vi "参数设置对画框.vi"(8 "时间等比采样":u16=10, 9 "单次采样量":u16=500, 10 "采样方式":enum16{"单采", "双重"}(ring), 11 "留样模式":T1(ring)=enum."外控留样") -> ()   [LabVIEW 2016, in "超标留样集成.lvlib" / "德润DR803L超标留样.lvlib"]
uses:
  <vilib>/Utility/config.llb/NI_LVConfig.lvlib
panel:
  in  "关闭":bool
  in  "打开串口":bool
  in  "释放串口":bool
  # "只在停止时切换有效"
  # "只在待机时切换有效"
  # "默认：500ml（5-1000）ml （只在停止时写有效）"
  # "默认：10min（2-9999）min （只在停止时写有效）"
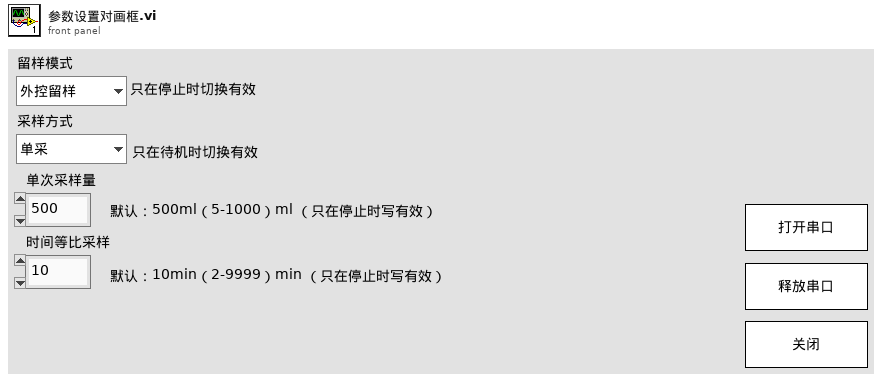
[diagram p1: front panel]
types:
  T1 = enum16{"无", "定时留样", "时间等比例", "超标留样", "同步留样", "外控留样"}
  T2 = enum16{"open", "read", "write", "write single", "close"}
  T3 = typedef "NI_LVConfig.lvlib/Config Data RefNum.ctl" = refnum<k1>
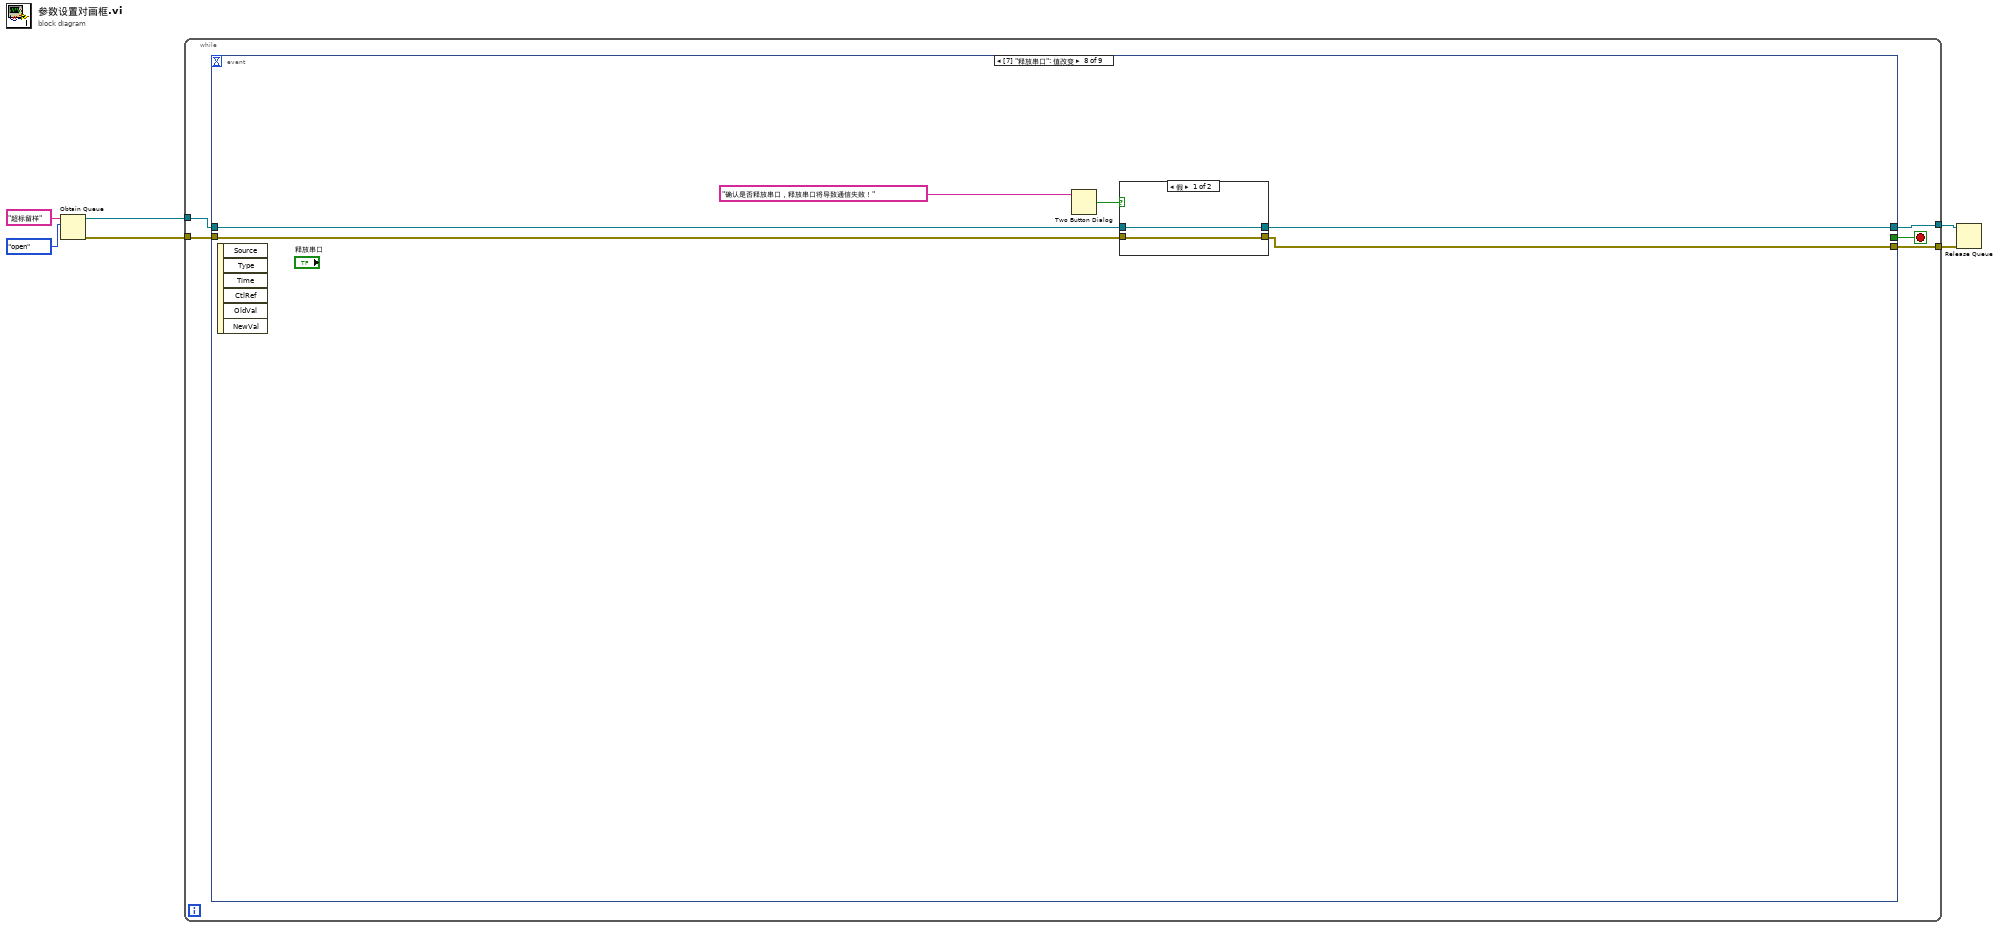
[diagram p0: block diagram]
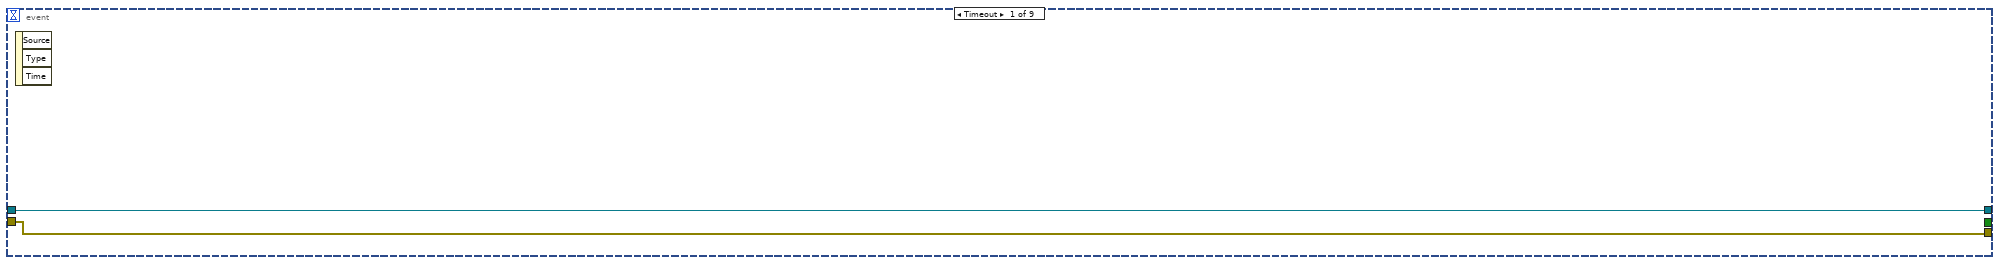
[diagram p2: hidden frame]
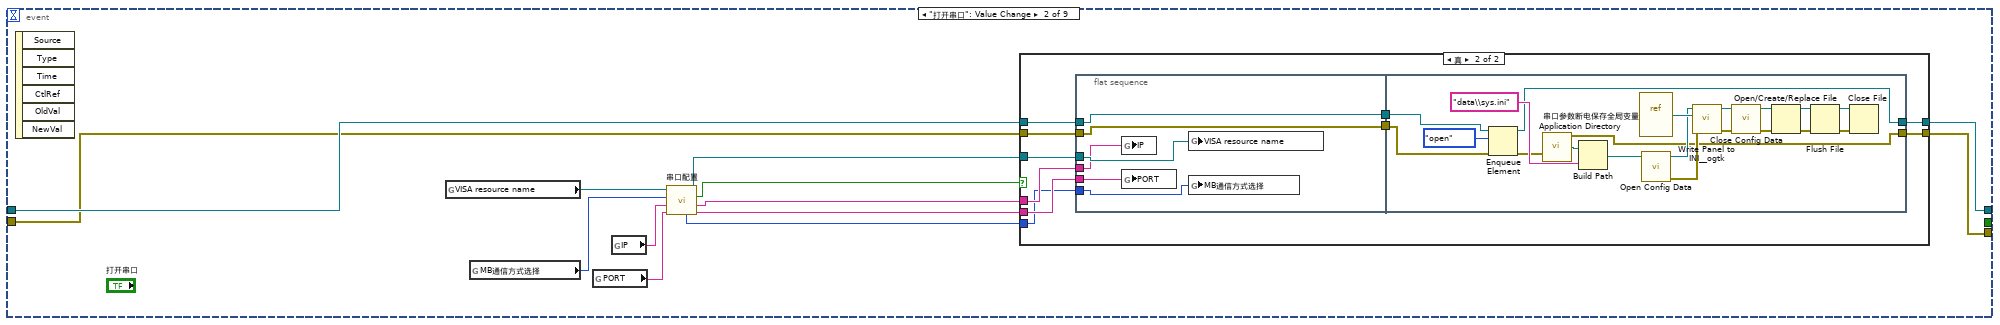
[diagram p3: hidden frame]
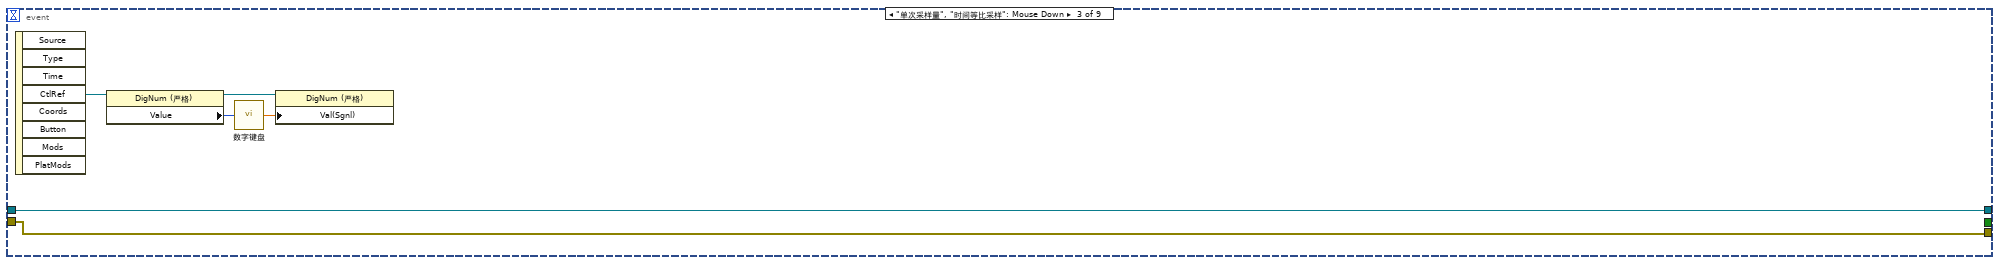
[diagram p5: hidden frame]
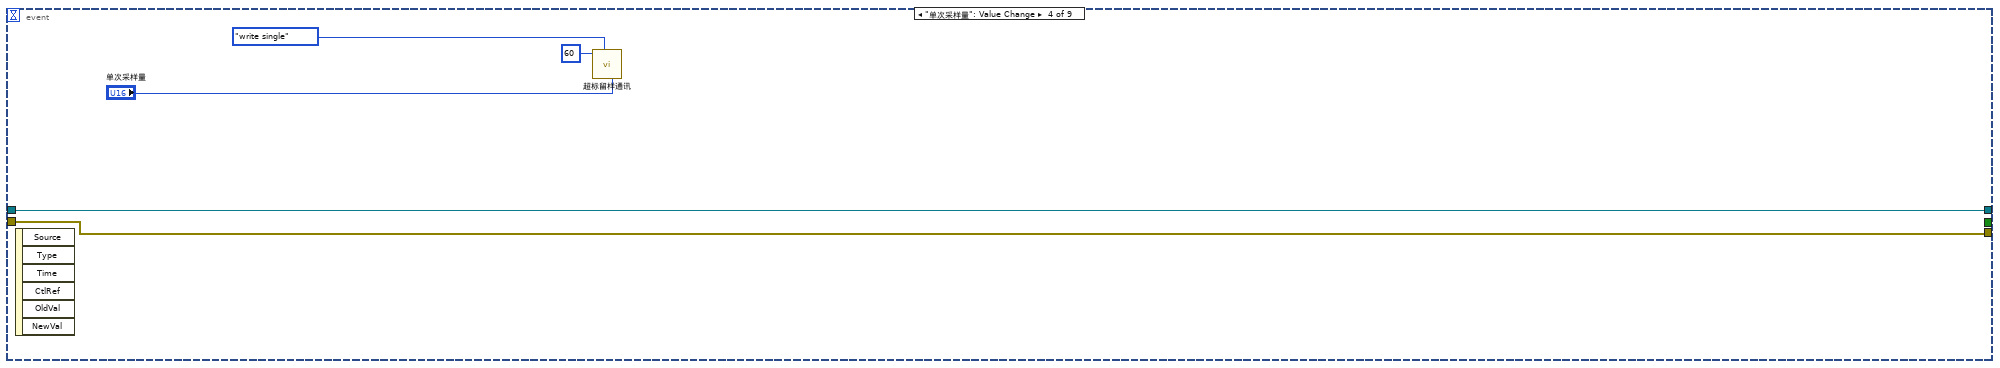
[diagram p6: hidden frame]
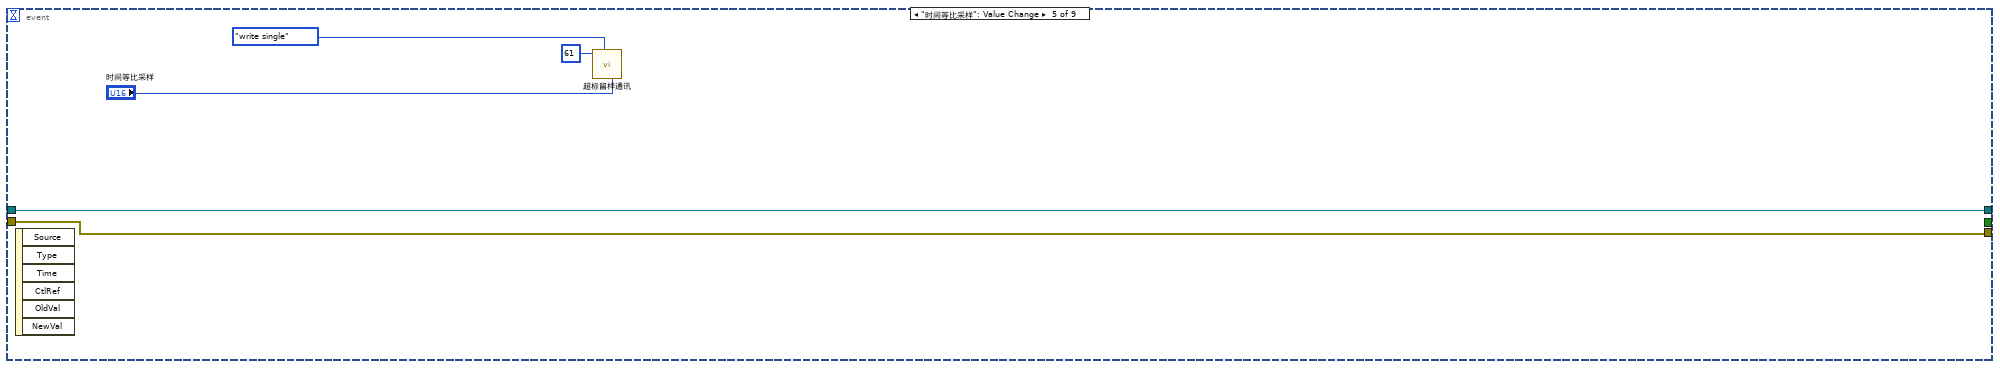
[diagram p7: hidden frame]
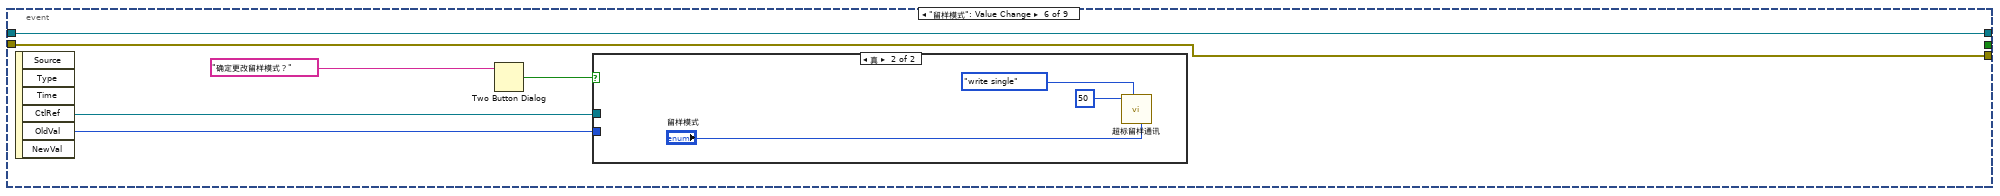
[diagram p8: hidden frame]
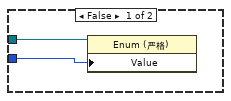
[diagram p9: hidden frame]
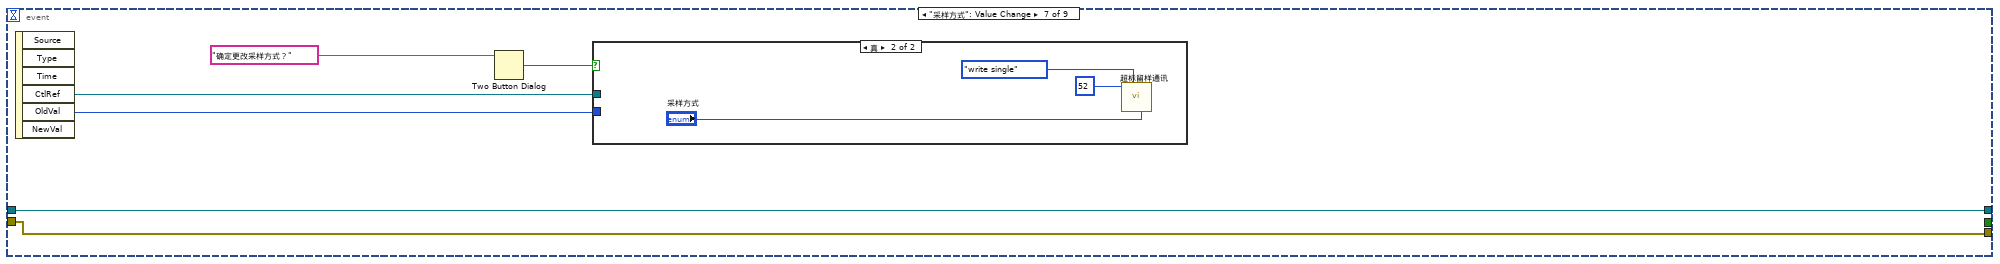
[diagram p10: hidden frame]
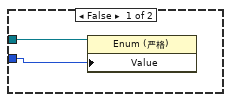
[diagram p11: hidden frame]
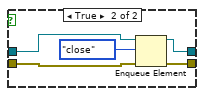
[diagram p12: hidden frame]
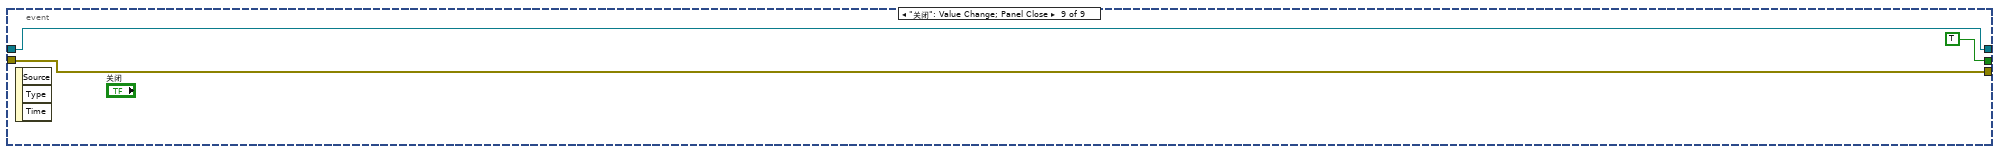
[diagram p13: hidden frame]
diagram:
  n1 = Obtain Queue(name (unnamed)="超标留样" ("名称（未命名）"), element data type=enum16{"open", "read", "write", "close"}."open") -> (queue out=w2:refnum<queue>, error out=w1:errorcluster)  [unwired: 3 in, 1 out]
  n2 = while {
    tunnel: w2 -> [w11]
    tunnel: w1 -> [w10]
    tunnel: [w9] -> w4
    tunnel: [w8] -> w3
    stop <- w7 stop-if-true
    n3 = event shown="[7] \"释放串口\": 值改变" {
      selector: _ -> [_ _ _ _ _ _ _ _ _]
      dyn-events: _ -> [_ _ _ _ _ _ _ _ _]
      timeout: _ -> [_ _ _ _ _ _ _ _ _]
      tunnel: w11 -> [w13 w17 w65 w71 w76 w81 w92 w105 w116]
      tunnel: w10 -> [w12 w16 w64 w70 w75 w80 w91 w104 w115]
      tunnel: [w13 w15 w65 w71 w76 w81 w92 w103 w116] -> w9
      tunnel: [w12 w14 w64 w70 w75 w80 w91 w102 w115] -> w8
      tunnel: [_ _ _ _ _ _ _ _ TRUE] -> w7
      event Timeout {
        n4 = event-data() -> ()  [unwired: 1 in, 3 out]
      }
      event "打开串口": Value Change {
        n5 = event-data() -> ()  [unwired: 1 in, 6 out]
        n6 = global read "串口参数断电保存全局变量.vi" "VISA resource name"() -> (w19:refnum<visa-resource-name>)
        n7 = global read "串口参数断电保存全局变量.vi" "MB通信方式选择"() -> (w18:enum16{"串口", "TCP"})
        n8 = global read "串口参数断电保存全局变量.vi" "PORT"() -> (w21:string)
        n9 = global read "串口参数断电保存全局变量.vi" "IP"() -> (w20:string)
        n10 = call "串口配置.vi"("PORT"=w21, "IP"=w20, "MB通信方式选择"=w18, "请选择串口:"=w19) -> ("PORT 2"=w25:string, "IP 2"=w24:string, "确认 2"=w22:bool, "VISA资源名称 2"=w23:refnum<visa-resource-name>, "MB通信方式选择 2"=w26:enum16{"串口", "TCP"})  [unwired: 3 in]
        n11 = case shown="真" w22 {
          tunnel: w23 -> [_ w38]
          tunnel: w24 -> [_ w37]
          tunnel: w25 -> [_ w36]
          tunnel: w26 -> [_ w35]
          tunnel: w17 -> [w28 w34]
          tunnel: w16 -> [w27 w32]
          tunnel: [w28 w30] -> w15
          tunnel: [w27 w29] -> w14
          frame False {
          }
          frame True {
            n12 = flat-sequence {
              tunnel: w38 -> [w44]
              tunnel: w37 -> [w43]
              tunnel: w36 -> [w42]
              tunnel: w35 -> [w41]
              tunnel: w34 -> [w40]
              tunnel: [w40] -> w33
              tunnel: w32 -> [w39]
              tunnel: [w39] -> w31
              tunnel: w33 -> [w48]
              tunnel: w31 -> [w47]
              tunnel: [w46] -> w30
              tunnel: [w45] -> w29
              frame #0 {
                n13 = global write "串口参数断电保存全局变量.vi" "IP"(w43) -> ()
                n14 = global write "串口参数断电保存全局变量.vi" "PORT"(w42) -> ()
                n15 = global write "串口参数断电保存全局变量.vi" "VISA resource name"(w44) -> ()
                n16 = global write "串口参数断电保存全局变量.vi" "MB通信方式选择"(w41) -> ()
              }
              frame #1 {
                n17 = Enqueue Element(queue=w48, element=enum16{"open", "read", "write", "close"}."open" ("元素"), error in (no error)=w47) -> (queue out=w46:refnum<queue>, error out=w45:errorcluster)  [unwired: 1 in, 1 out]
                n18 = call <vilib>:"Application Directory.vi"() -> ("Application Directory"=w51:path)
                n19 = Build Path(base path=w51, name or relative path="data\\sys.ini" ("名称或相对路径")) -> (appended path=w52:path)
                n20 = vi-ref "串口参数断电保存全局变量.vi"() -> (w54:refnum<vi>)
                n21 = call <vilib>:"Open Config Data.vi"("configuration file path"=w52) -> ("error out"=w56:errorcluster, "refnum"=w53:T3)  [unwired: 8 in, 1 out]
                n22 = call <userlib>:"Write Panel to INI__ogtk.vi"("error in (no error)"=w56, "VI ref"=w54, "refnum"=w53) -> ("error out"=w57:errorcluster, "refnum out"=w55:T3)  [unwired: 7 in]
                n23 = call <vilib>:"Close Config Data.vi"("error in (no error)"=w57, "refnum"=w55) -> ("error out"=w62:errorcluster, "file path"=w63:path)  [unwired: 8 in]
                n24 = Open/Create/Replace File(file path (use dialog)=w63, error in=w62) -> (refnum out=w59:refnum<file>, error out=w58:errorcluster)  [unwired: 4 in, 1 out]
                n25 = Flush File(refnum=w59, error in=w58) -> (refnum out=w60:refnum<file>, error out=w61:errorcluster)
                n26 = Close File(refnum=w60, error in=w61) -> ()  [unwired: 2 out]
              }
            }
          }
        }
      }
      event "单次采样量", "时间等比采样": Mouse Down {
        n27 = event-data() -> ("CtlRef"=w66:refnum<vi>)  [unwired: 1 in, 7 out]
        n28 = property class="DigNum (严格)"(reference=w66) -> (reference out=w69:refnum<vi>, "Value"=w68:u16)  [unwired: 1 in, 1 out]
        n29 = call "数字键盘.vi"("OldNumber"=w68) -> ("NewNumber"=w67:sgl)
        n30 = property class="DigNum (严格)"(reference=w69, "Val(Sgnl)"=w67) -> ()  [unwired: 1 in, 2 out]
      }
      event "单次采样量": Value Change {
        n31 = event-data() -> ()  [unwired: 1 in, 6 out]
        n32 = call "超标留样通讯.vi"("value"="单次采样量", "STEP"=T2."write single", "starting address"=60 ("索引")) -> ()  [unwired: 6 in, 3 out]
      }
      event "时间等比采样": Value Change {
        n33 = event-data() -> ()  [unwired: 1 in, 6 out]
        n34 = call "超标留样通讯.vi"("value"="时间等比采样", "STEP"=T2."write single", "starting address"=61 ("索引")) -> ()  [unwired: 6 in, 3 out]
      }
      event "留样模式": Value Change {
        n35 = event-data() -> ("CtlRef"=w83:refnum<vi>, "OldVal"=w82:T1)  [unwired: 1 in, 4 out]
        n36 = Two Button Dialog(message="确定更改留样模式？" ("消息")) -> (T button?=w84:bool)  [unwired: 2 in]
        n37 = case shown="真" w84 {
          tunnel: w82 -> [w86 _]
          tunnel: w83 -> [w87 _]
          frame False {
            n38 = property class="Enum (严格)"(reference=w87, "Value"=w86) -> ()  [unwired: 1 in, 2 out]
          }
          frame True {
            n39 = call "超标留样通讯.vi"("value"="留样模式", "STEP"=T2."write single", "starting address"=50 ("索引")) -> ()  [unwired: 6 in, 3 out]
          }
        }
      }
      event "采样方式": Value Change {
        n40 = event-data() -> ("CtlRef"=w94:refnum<vi>, "OldVal"=w93:enum16{"单采", "双重"})  [unwired: 1 in, 4 out]
        n41 = Two Button Dialog(message="确定更改采样方式？" ("消息")) -> (T button?=w95:bool)  [unwired: 2 in]
        n42 = case shown="真" w95 {
          tunnel: w94 -> [w98 _]
          tunnel: w93 -> [w97 _]
          frame False {
            n43 = property class="Enum (严格)"(reference=w98, "Value"=w97) -> ()  [unwired: 1 in, 2 out]
          }
          frame True {
            n44 = call "超标留样通讯.vi"("value"="采样方式", "STEP"=T2."write single", "starting address"=52 ("索引")) -> ()  [unwired: 6 in, 3 out]
          }
        }
      }
      event "释放串口": Value Change {
        n45 = event-data() -> ()  [unwired: 1 in, 6 out]
        n46 = Two Button Dialog(message="确认是否释放串口，释放串口将导致通信失败！" ("消息")) -> (T button?=w106:bool)  [unwired: 2 in]
        n47 = case shown="假" w106 {
          tunnel: w105 -> [w109 w113]
          tunnel: w104 -> [w108 w112]
          tunnel: [w109 w111] -> w103
          tunnel: [w108 w110] -> w102
          frame False {
          }
          frame True {
            n48 = Enqueue Element(queue=w113, element=enum16{"open", "read", "write", "close"}."close" ("元素"), error in (no error)=w112) -> (queue out=w111:refnum<queue>, error out=w110:errorcluster)  [unwired: 1 in, 1 out]
          }
        }
      }
      event "关闭": Value Change; Panel Close {
        n49 = event-data() -> ()  [unwired: 1 in, 3 out]
      }
    }
  }
  n50 = Release Queue(queue=w4, error in (no error)=w3) -> ()  [unwired: 1 in, 3 out]
